vi "Bounds.vi"(8 "Low":dbl=3.0, 9 "Hight":dbl=4.0, 11 "N":dbl) -> (3 "Res":dbl)   [LabVIEW 2023]
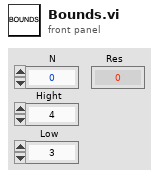
[diagram p1: front panel]
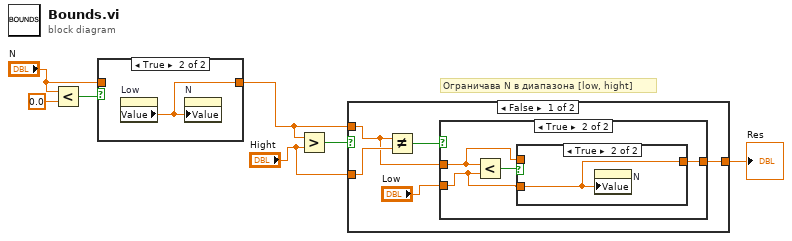
[diagram p0: block diagram]
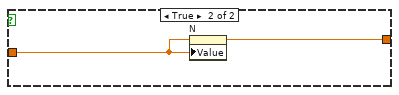
[diagram p5: hidden frame]
diagram:
  # "Ограничава N в диапазона [low, hight]"
  n1 = Less?(x="N", y=0.0) -> (x < y?=w4:bool)
  n2 = case shown="True" w4 {
    tunnel: [w8 w9] -> w3
    tunnel: "N" -> [w8 _]
    frame False {
    }
    frame True {
      n3 = property on="Low" class="DigNum (strict)"() -> ("Value"=w9:dbl)  [unwired: 2 in, 2 out]
      n4 = property on="N" class="DigNum (strict)"("Value"=w9) -> ()  [unwired: 2 in, 2 out]
    }
  }
  n5 = Greater?(x=w3, y="Hight") -> (0:w7:bool)
  n6 = case shown="False" w7 {
    tunnel: w3 -> [w12 _]
    tunnel: "Hight" -> [w14 w22]
    tunnel: [w10 w22] -> w1
    frame False {
      n7 = Not Equal?(x=w12, y=w14) -> (x != y?=w13:bool)
      n8 = case shown="True" w13 {
        tunnel: w12 -> [w15 w16]
        tunnel: "Low" -> [_ w17]
        tunnel: [w15 w18] -> w10
        frame False {
        }
        frame True {
          n9 = Less?(x=w16, y=w17) -> (x < y?=w19:bool)
          n10 = case shown="True" w19 {
            tunnel: w17 -> [_ w21]
            tunnel: [w20 w21] -> w18
            tunnel: w16 -> [w20 _]
            frame False {
            }
            frame True {
              n11 = property on="N" class="DigNum (strict)"("Value"=w21) -> ()  [unwired: 2 in, 2 out]
            }
          }
        }
      }
    }
    frame True {
      n12 = property on="N" class="DigNum (strict)"("Value"=w22) -> ()  [unwired: 2 in, 2 out]
    }
  }
  "Res" <- w1
